vi "Make Receiver.vi"(8 "error in (no error)":errorcluster, 11 "Coupled Message Scripter in":refnum<class "Coupled Message Scripter.lvclass">) -> (0 "error out":errorcluster, 3 "Coupled Message Scripter out":refnum<class "Coupled Message Scripter.lvclass">)   [LabVIEW 2020, in "Message Maker.lvlib" / "Coupled Message Scripter.lvclass"]
uses:
  Coupled Message Scripter.lvclass
  Message Maker.lvlib
  Message Scripter/Message Scripter.lvclass
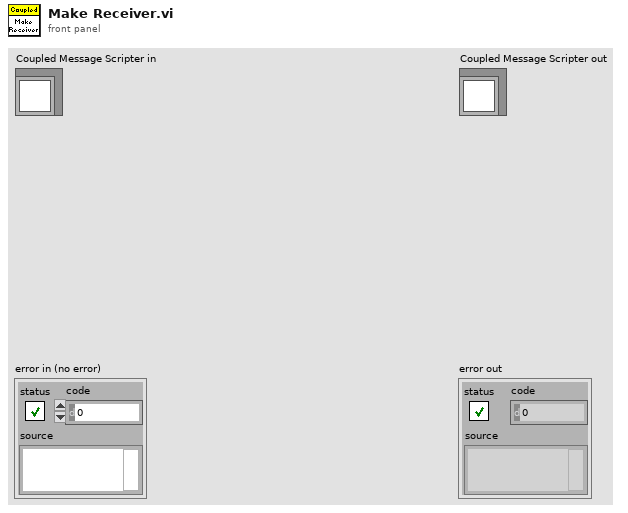
[diagram p1: front panel]
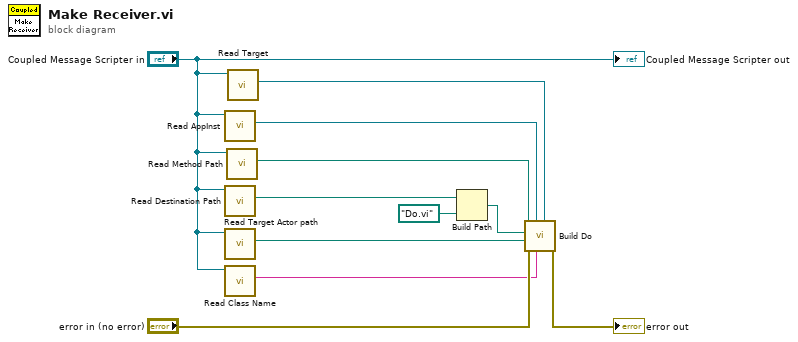
[diagram p0: block diagram]
diagram:
  n1 = call "Read AppInst.vi"("Message Maker in"="Coupled Message Scripter in") -> ("AppInst"=w5:refnum<vi>)  [unwired: 10 in]
  n2 = call "Read Destination Path.vi"("Message Scripter in"="Coupled Message Scripter in") -> ("Destination Path"=w9:path)  [unwired: 10 in]
  n3 = call "Read Target Actor path.vi"("Message Scripter in"="Coupled Message Scripter in") -> ("Target Actor path"=w4:path)  [unwired: 10 in]
  n4 = call "Read Class Name.vi"("Message Scripter in"="Coupled Message Scripter in") -> ("Class Name"=w6:string)  [unwired: 10 in]
  n5 = call "Read Method Path.vi"("Message Maker in"="Coupled Message Scripter in") -> ("Method Path"=w3:path)  [unwired: 10 in]
  n6 = call "Read Target.vi"("Message Scripter in"="Coupled Message Scripter in") -> ("Target"=w1:refnum<vi>)  [unwired: 10 in]
  n7 = Build Path(base path=w9, name or relative path=path "Do.vi") -> (appended path=w11:path)
  n8 = call "Build Do.vi"("Target"=w1, "Class Name"=w6, "AppInst"=w5, "error in (no error)"="error in (no error)", "Actor class path"=w4, "Do Method path"=w11, "Target Method path"=w3) -> ("error out"=→"error out":errorcluster)  [unwired: 4 in]
  "Coupled Message Scripter out" <- "Coupled Message Scripter in"
